vi "MCL Volts Transactions List.vi"() -> (2 "Transactions":string[](array[string]))   [LabVIEW 2013]
uses:
  Names/Source Group Type.ctl
panel:
  in  "Sources":T1[](array[typedef])=[enum."LBCB1", enum."LBCB2"]
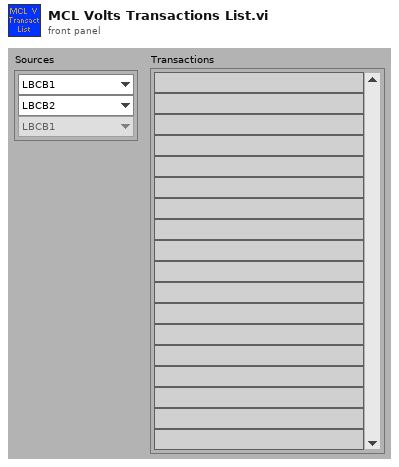
[diagram p1: front panel]
types:
  T1 = typedef "Source Group Type.ctl" = enum16{"LBCB1", "LBCB2", "Consolidated", "External"}
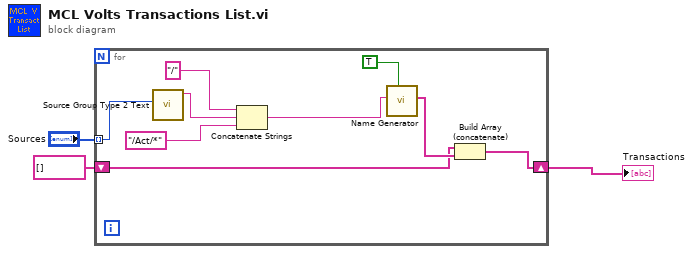
[diagram p0: block diagram]
diagram:
  n1 = for {
    tunnel: "Sources" -> [w12] mode=indexing
    shift-right: [w6] -> w2
    shift-left: string[] [] -> [w5]
    n2 = call "Source Group Type 2 Text.vi"("Source"=w12) -> ("String"=w11:string)  [unwired: 10 in]
    n3 = Concatenate Strings("/" ("string"), w11, "/Act/*" ("string")) -> (w8:string)
    n4 = call "Name Generator.vi"("Keep Servo Error"=TRUE, "Group Specifier"=w8) -> ("Group Names"=w7:string[])  [unwired: 9 in]
    n5 = Build Array (concatenate)(w5, w7) -> (w6:string[])
  }
  "Transactions" <- w2
